vi "16进制字符转16进制数字.vi"(11 "data in":string) -> (3 "number":u32 format="%x")   [LabVIEW 2017]
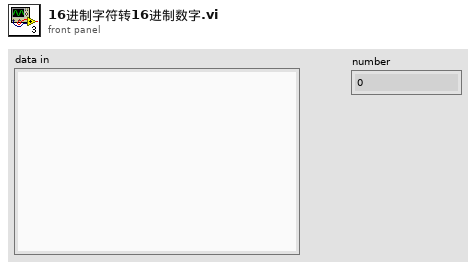
[diagram p1: front panel]
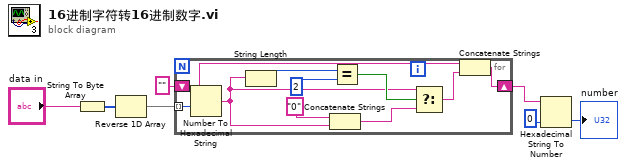
[diagram p0: block diagram]
diagram:
  n1 = String To Byte Array(string="data in") -> (unsigned byte array=w3:u8[])
  n2 = Reverse 1D Array(array=w3) -> (reversed array=w1:u8[])
  n3 = for {
    shift-right: [w16] -> w5
    shift-left: "" ("format string") -> [w8]
    tunnel: w1 -> [w17] mode=indexing
    n4 = Number To Hexadecimal String(2:w17) -> (0:w10:string)  [unwired: 1 in]
    n5 = String Length(string=w10) -> (length=w15:i32)
    n6 = Concatenate Strings("0" ("format string"), w10) -> (w12:string)
    n7 = Equal?(x=w15, y=2) -> (x = y?=w13:bool)
    n8 = Select(t=w10, s=w13, f=w12) -> (s? t:f=w9:string)
    n9 = Concatenate Strings(w8, w9) -> (w16:string)
  }
  n10 = Hexadecimal String To Number(string=w5, default (0uL)=u64 0 ("default (0 U32)")) -> (number=→"number":u64)  [unwired: 1 in, 1 out]
